vi "Read Video.vi"(6 "error in (no error)":errorcluster, 9 "input cluster":T6={"Video Resolution"=enum."FREENECT_RESOLUTION_LOW", "Video Format"=enum."FREENECT_VIDEO_RGB", "Depth Format"=enum."FREENECT_DEPTH_11BIT", "Depth Resolution"=enum."FREENECT_RESOLUTION_LOW"}) -> (0 "error out":errorcluster, 1 "raw data":u32[][](array[numeric]), 2 "Distance O":dbl, 3 "RGB image":picture, 4 "y":dbl, 5 "x":dbl)   [LabVIEW 2015]
uses:
  Video Resolution Control.ctl
  Video Format Control.ctl
  Depth Resolution Control.ctl
  <vilib>/picture/picture.llb/Draw True-Color Pixmap.vi
  libkinect_wrapper.dll
  <vilib>/vision/NI_Vision_Development_Module.lvlib
panel:
  out "Distance H":dbl
  out "Width":dbl
  in  "Number of Erosion":i32=2
  out "Centroid":cluster{"X Centroid":sgl, "Y Centroid":sgl} {"Y Centroid" format="%.2f"; "X Centroid" format="%.2f"}
  out "Largest Particle Image":T1(plugin-control)
  in  "HSL Ranges":T2={"Hue Range"={"Lower value"=80, "Upper value"=255}, "Sat Range"={"Lower value"=0, "Upper value"=30}, "Luma Range"={"Lower value"=0, "Upper value"=60}}
  out "error out 3":errorcluster
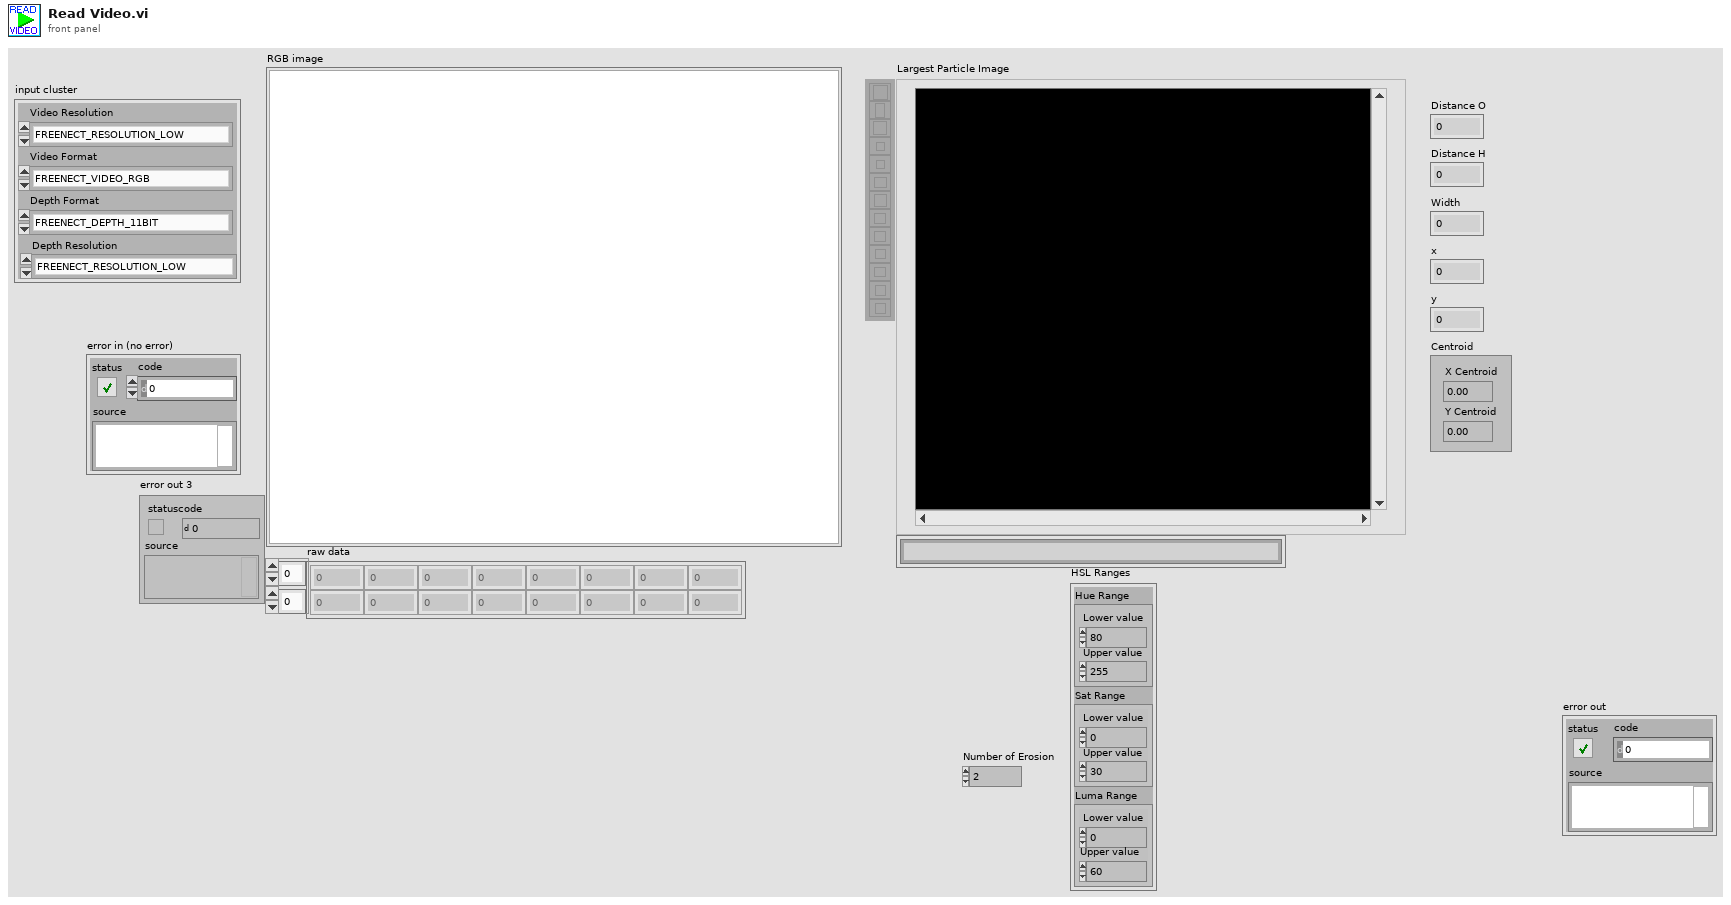
[diagram p1: front panel]
types:
  T1 = typedef "IMAQ Image.ctl" = refnum<image>
  T2 = cluster{"Hue Range":cluster{"Lower value":i32, "Upper value":i32}, "Sat Range":cluster{"Lower value":i32, "Upper value":i32}, "Luma Range":cluster{"Lower value":i32, "Upper value":i32}}
  T3 = typedef "Video Resolution Control.ctl" = enum32{"FREENECT_RESOLUTION_LOW", "FREENECT_RESOLUTION_MEDIUM", "FREENECT_RESOLUTION_HIGH"}
  T4 = typedef "Video Format Control.ctl" = enum32{"FREENECT_VIDEO_RGB", "FREENECT_VIDEO_BAYER", "FREENECT_VIDEO_IR_8BIT", "FREENECT_VIDEO_IR_10BIT", "FREENECT_VIDEO_IR_10BIT_PACKED", "FREENECT_VIDEO_YUV_RGB", "FREENECT_VIDEO_YUV_RAW"}
  T5 = typedef "Depth Resolution Control.ctl" = enum16{"FREENECT_RESOLUTION_TINY", "FREENECT_RESOLUTION_LOW", "FREENECT_RESOLUTION_MEDIUM"}
  T6 = cluster{"Video Resolution":T3, "Video Format":T4, "Depth Format":enum32{"FREENECT_DEPTH_11BIT", "FREENECT_DEPTH_10BIT", "FREENECT_DEPTH_11BIT_PACKED", "FREENECT_DEPTH_10BIT_PACKED", "FREENECT_DEPTH_REGISTERED", "FREENECT_DEPTH_MM"}, "Depth Resolution":T5}
  T7 = cluster{"X Size":i32, "Y Size":i32, "Order #":i32}
  T8 = typedef "Image Type" = u32
  T9 = cluster{"Area":dbl, "Number of Holes":dbl, "Bounding Rect":cluster{"Left":dbl, "Top":dbl, "Right":dbl, "Bottom":dbl}, "Center of Mass":cluster{"X":dbl, "Y":dbl}, "Orientation":dbl, "Dimensions":cluster{"Width":dbl, "Height":dbl}}[]
  T10 = cluster{"Area":dbl, "Number of Holes":dbl, "Bounding Rect":cluster{"Left":dbl, "Top":dbl, "Right":dbl, "Bottom":dbl}, "Center of Mass":cluster{"X":dbl, "Y":dbl}, "Orientation":dbl, "Dimensions":cluster{"Width":dbl, "Height":dbl}}
  T11 = cluster{"Left":dbl, "Top":dbl, "Right":dbl, "Bottom":dbl}
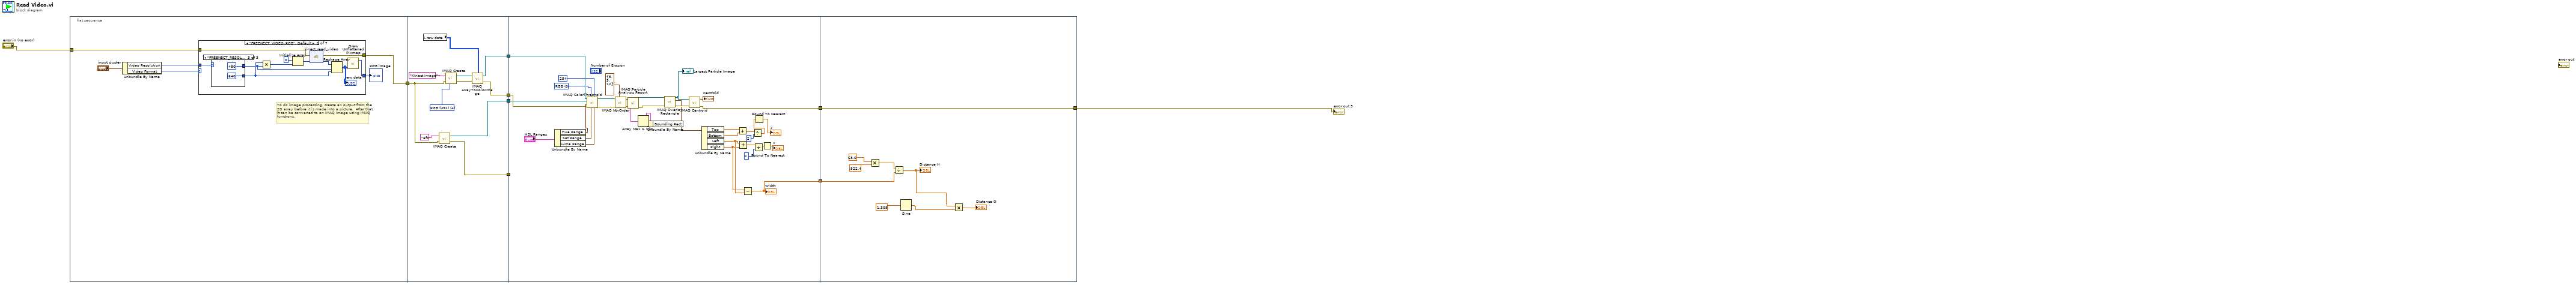
[diagram p0: block diagram]
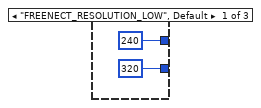
[diagram p2: hidden frame]
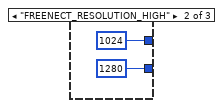
[diagram p3: hidden frame]
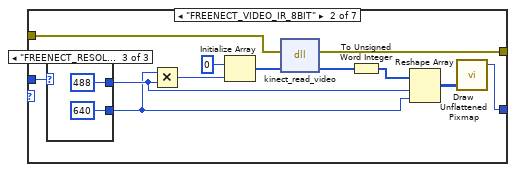
[diagram p4: hidden frame]
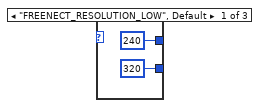
[diagram p5: hidden frame]
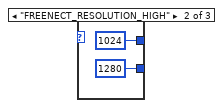
[diagram p6: hidden frame]
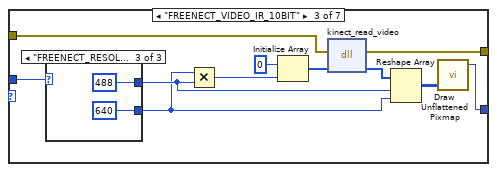
[diagram p7: hidden frame]
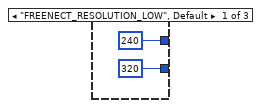
[diagram p8: hidden frame]
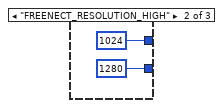
[diagram p9: hidden frame]
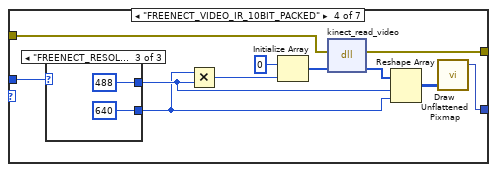
[diagram p10: hidden frame]
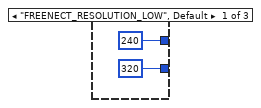
[diagram p11: hidden frame]
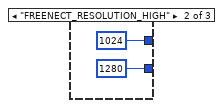
[diagram p12: hidden frame]
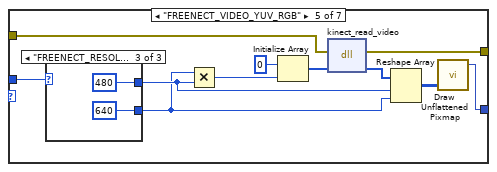
[diagram p13: hidden frame]
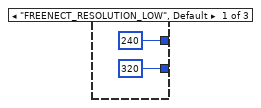
[diagram p14: hidden frame]
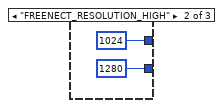
[diagram p15: hidden frame]
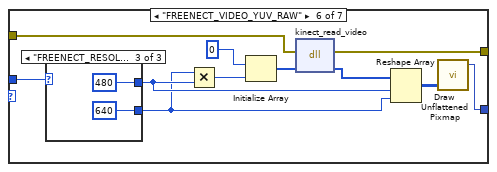
[diagram p16: hidden frame]
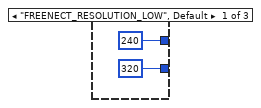
[diagram p17: hidden frame]
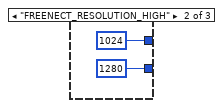
[diagram p18: hidden frame]
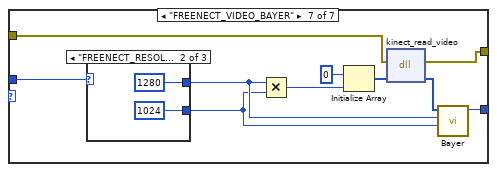
[diagram p19: hidden frame]
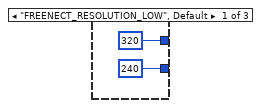
[diagram p20: hidden frame]
diagram:
  n1 = flat-sequence {
    tunnel: [w12] -> w9
    tunnel: "error in (no error)" -> [w10]
    tunnel: w9 -> [w136]
    tunnel: [w143] -> w7
    tunnel: [w140] -> w6
    tunnel: [w138] -> w5
    tunnel: [w135] -> w3
    tunnel: w7 -> [w168]
    tunnel: w6 -> [w157]
    tunnel: w5 -> [w169]
    tunnel: [w173] -> w4
    tunnel: w3 -> [_]
    tunnel: [w150] -> w1
    tunnel: w4 -> [w190]
    tunnel: [w190] -> w2
    tunnel: w1 -> [w186]
    frame #0 {
      # "To do image processing, create an output from the 2D array before it is made into a picture.  After that, it can be converted to an IMAQ image using IMAQ functions."
      n2 = Unbundle By Name("input cluster") -> ("Video Resolution"=w13:T3, "Video Format"=w14:T4)
      n3 = case shown="\"FREENECT_VIDEO_RGB\", Default" w14 {
        tunnel: w13 -> [w26 w36 w51 w70 w95 w112 w121]
        tunnel: [w22 w38 w53 w72 w89 w103 w122] -> w11
        tunnel: w10 -> [w21 w37 w52 w71 w88 w108 w124]
        tunnel: [w20 w39 w54 w73 w87 w107 w123] -> w12
        frame "FREENECT_VIDEO_RGB", Default {
          n4 = case shown="\"FREENECT_RESOLUTION_MEDIUM\"" w26 {
            tunnel: [240 1024 480] -> w19
            tunnel: [320 1280 640] -> w18
            frame "FREENECT_RESOLUTION_LOW", Default {
            }
            frame "FREENECT_RESOLUTION_HIGH" {
            }
            frame "FREENECT_RESOLUTION_MEDIUM" {
            }
          }
          n5 = Multiply(x=w18, y=w19) -> (x*y=w25:i32)
          n6 = Initialize Array(u32 0 ("U32"), w25) -> (w24:u32[])
          n7 = dll-call lib="libkinect_wrapper.*" fn="kinect_read_video"(error in=w21, "video"=w24) -> (error out=w20:errorcluster, "video"=w17:u32[])  [unwired: 3 in, 1 out]
          n8 = Reshape Array(w17, w19, w18) -> (w16:u32[][])
          "raw data" <- w16
          n9 = call-poly <vilib>:"Draw Unflattened Pixmap.vi"("data (RGB format)"=w16) -> ("new picture"=w22:picture)  [unwired: 8 in]
        }
        frame "FREENECT_VIDEO_IR_8BIT" {
          n10 = case shown="\"FREENECT_RESOLUTION_MEDIUM\"" w36 {
            tunnel: [240 1024 488] -> w41
            tunnel: [320 1280 640] -> w40
            frame "FREENECT_RESOLUTION_LOW", Default {
            }
            frame "FREENECT_RESOLUTION_HIGH" {
            }
            frame "FREENECT_RESOLUTION_MEDIUM" {
            }
          }
          n11 = Multiply(x=w40, y=w41) -> (x*y=w44:i32)
          n12 = Initialize Array(u8 0 ("U32"), w44) -> (w43:u8[])
          n13 = dll-call lib="libkinect_wrapper.*" fn="kinect_read_video"(error in=w37, "video"=w43) -> (error out=w39:errorcluster, "video"=w35:u8[])  [unwired: 3 in, 1 out]
          n14 = To Unsigned Word Integer(number=w35) -> (unsigned 16bit integer=w34:u16[])
          n15 = Reshape Array(w34, w41, w40) -> (w33:u16[][])
          n16 = call-poly <vilib>:"Draw Unflattened Pixmap.vi"("data (RGB format)"=w33) -> ("new picture"=w38:picture)  [unwired: 8 in]
        }
        frame "FREENECT_VIDEO_IR_10BIT" {
          n17 = case shown="\"FREENECT_RESOLUTION_MEDIUM\"" w51 {
            tunnel: [240 1024 488] -> w56
            tunnel: [320 1280 640] -> w55
            frame "FREENECT_RESOLUTION_LOW", Default {
            }
            frame "FREENECT_RESOLUTION_HIGH" {
            }
            frame "FREENECT_RESOLUTION_MEDIUM" {
            }
          }
          n18 = Multiply(x=w55, y=w56) -> (x*y=w61:i32)
          n19 = Initialize Array(u16 0 ("U32"), w61) -> (w60:u16[])
          n20 = dll-call lib="libkinect_wrapper.*" fn="kinect_read_video"(error in=w52, "video"=w60) -> (error out=w54:errorcluster, "video"=w58:u16[])  [unwired: 3 in, 1 out]
          n21 = Reshape Array(w58, w56, w55) -> (w57:u16[][])
          n22 = call-poly <vilib>:"Draw Unflattened Pixmap.vi"("data (RGB format)"=w57) -> ("new picture"=w53:picture)  [unwired: 8 in]
        }
        frame "FREENECT_VIDEO_IR_10BIT_PACKED" {
          n23 = case shown="\"FREENECT_RESOLUTION_MEDIUM\"" w70 {
            tunnel: [240 1024 488] -> w75
            tunnel: [320 1280 640] -> w74
            frame "FREENECT_RESOLUTION_LOW", Default {
            }
            frame "FREENECT_RESOLUTION_HIGH" {
            }
            frame "FREENECT_RESOLUTION_MEDIUM" {
            }
          }
          n24 = Multiply(x=w74, y=w75) -> (x*y=w78:i32)
          n25 = Initialize Array(u16 0 ("U32"), w78) -> (w77:u16[])
          n26 = dll-call lib="libkinect_wrapper.*" fn="kinect_read_video"(error in=w71, "video"=w77) -> (error out=w73:errorcluster, "video"=w69:u16[])  [unwired: 3 in, 1 out]
          n27 = Reshape Array(w69, w75, w74) -> (w68:u16[][])
          n28 = call-poly <vilib>:"Draw Unflattened Pixmap.vi"("data (RGB format)"=w68) -> ("new picture"=w72:picture)  [unwired: 8 in]
        }
        frame "FREENECT_VIDEO_YUV_RGB" {
          n29 = case shown="\"FREENECT_RESOLUTION_MEDIUM\"" w95 {
            tunnel: [240 1024 480] -> w86
            tunnel: [320 1280 640] -> w85
            frame "FREENECT_RESOLUTION_LOW", Default {
            }
            frame "FREENECT_RESOLUTION_HIGH" {
            }
            frame "FREENECT_RESOLUTION_MEDIUM" {
            }
          }
          n30 = Multiply(x=w85, y=w86) -> (x*y=w94:i32)
          n31 = Initialize Array(u32 0 ("U32"), w94) -> (w93:u32[])
          n32 = dll-call lib="libkinect_wrapper.*" fn="kinect_read_video"(error in=w88, "video"=w93) -> (error out=w87:errorcluster, "video"=w91:u32[])  [unwired: 3 in, 1 out]
          n33 = Reshape Array(w91, w86, w85) -> (w90:u32[][])
          n34 = call-poly <vilib>:"Draw Unflattened Pixmap.vi"("data (RGB format)"=w90) -> ("new picture"=w89:picture)  [unwired: 8 in]
        }
        frame "FREENECT_VIDEO_YUV_RAW" {
          n35 = case shown="\"FREENECT_RESOLUTION_MEDIUM\"" w112 {
            tunnel: [240 1024 480] -> w106
            tunnel: [320 1280 640] -> w105
            frame "FREENECT_RESOLUTION_LOW", Default {
            }
            frame "FREENECT_RESOLUTION_HIGH" {
            }
            frame "FREENECT_RESOLUTION_MEDIUM" {
            }
          }
          n36 = Multiply(x=w105, y=w106) -> (x*y=w111:i32)
          n37 = Initialize Array(u16 0 ("U32"), w111) -> (w110:u16[])
          n38 = dll-call lib="libkinect_wrapper.*" fn="kinect_read_video"(error in=w108, "video"=w110) -> (error out=w107:errorcluster, "video"=w104:u16[])  [unwired: 3 in, 1 out]
          n39 = Reshape Array(w104, w106, w105) -> (w102:u16[][])
          n40 = call-poly <vilib>:"Draw Unflattened Pixmap.vi"("data (RGB format)"=w102) -> ("new picture"=w103:picture)  [unwired: 8 in]
        }
        frame "FREENECT_VIDEO_BAYER" {
          n41 = case shown="\"FREENECT_RESOLUTION_HIGH\"" w121 {
            tunnel: [320 1280 640] -> w120
            tunnel: [240 1024 480] -> w119
            frame "FREENECT_RESOLUTION_LOW", Default {
            }
            frame "FREENECT_RESOLUTION_HIGH" {
            }
            frame "FREENECT_RESOLUTION_MEDIUM" {
            }
          }
          n42 = Multiply(x=w120, y=w119) -> (x*y=w128:i32)
          n43 = Initialize Array(u8 0, w128) -> (w127:u8[])
          n44 = dll-call lib="libkinect_wrapper.*" fn="kinect_read_video"(error in=w124, "video"=w127) -> (error out=w123:errorcluster, "video"=w126:u8[])  [unwired: 3 in, 1 out]
          n45 = call "Bayer.vi"("Height"=w119, "Width"=w120, "Array"=w126) -> ("new picture"=w122:picture)  [unwired: 8 in]
        }
      }
      "RGB image" <- w11
    }
    frame #1 {
      w137 = T8 4 items=["Grayscale (U8)", "Grayscale (I16)", "Grayscale (SGL)", "Complex (CSG)", "RGB (U32)", "HSL (U32)", "RGB (U64)", "Grayscale (U16)"] ("Image Type")
      n46 = local read "raw data"() -> (w141:u32[][])
      n47 = call "IMAQ Create"("Image Name"="afs", "error in (no error)"=w136) -> ("New Image"=w138:T1, "error out"=w135:errorcluster)  [unwired: 3 in]
      n48 = call "IMAQ Create"("Image Name"="Kinect image", "Image Type"=w137, "error in (no error)"=w136) -> ("New Image"=w145:T1, "error out"=w144:errorcluster)  [unwired: 2 in]
      n49 = call "IMAQ ArrayToColorImage"("Image Pixels (U32)"=w141, "Image"=w145, "error in (no error)"=w144) -> ("Image Out"=w140:T1, "error out"=w143:errorcluster)  [unwired: 2 in]
    }
    frame #2 {
      w170 = u16 0 items=["RGB", "HSL", "HSV", "HSI"] ("Color Mode")
      n50 = Unbundle By Name("HSL Ranges") -> ("Hue Range"=w180:cluster{"Lower value":i32, "Upper value":i32}, "Sat Range"=w179:cluster{"Lower value":i32, "Upper value":i32}, "Luma Range"=w158:cluster{"Lower value":i32, "Upper value":i32})
      n51 = call "IMAQ ColorThreshold"("Blue or Luma or Val or Inten Range"=w158, "Replace Value"=254, "Green or Sat Range"=w179, "Color Mode"=w170, "error in (no error)"=w168, "Red or Hue Range"=w180, "Image Dst"=w169, "Image Src"=w157) -> ("error out"=w146:errorcluster, "Image Dst Out"=w147:T1)  [unwired: 2 in]
      n52 = call "IMAQ NthOrder"("Image Src"=w147, "Size & Order #"=T7 {"X Size"=5, "Y Size"=5, "Order #"=12}, "error in (no error)"=w146) -> ("Image Dst Out"=w155:T1, "error out"=w154:errorcluster)  [unwired: 4 in]
      n53 = call "IMAQ Particle Analysis Report"("error in (no error)"=w154, "Image"=w155) -> ("error out"=w176:errorcluster, "Particle Reports (Pixels)"=w177:T9, "Image Out (duplicate)"=w156:T1)  [unwired: 4 in, 3 out]
      n54 = Array Max & Min(array=w177) -> (max value=w175:T10)  [unwired: 3 out]
      n55 = Unbundle By Name(w175) -> ("Bounding Rect"=w167:T11)
      n56 = call "IMAQ Overlay Rectangle"("error in (no error)"=w176, "Rectangle"=w167, "Image"=w156) -> ("error out"=w174:errorcluster, "Image Out"=w172:T1)  [unwired: 7 in]
      "Largest Particle Image" <- w172
      n57 = call "IMAQ Centroid"("error in (no error)"=w174, "Image"=w172) -> ("error out"=w173:errorcluster, "Centroid"=→"Centroid":cluster{"X Centroid":sgl, "Y Centroid":sgl})  [unwired: 2 in]
      n58 = Unbundle By Name(w167) -> ("Top"=w149:dbl, "Bottom"=w148:dbl, "Left"=w152:dbl, "Right"=w151:dbl)
      n59 = Add(x=w149, y=w148) -> (x+y=w165:dbl)
      n60 = Add(x=w152, y=w151) -> (x+y=w166:dbl)
      n61 = Subtract(x=w151, y=w152) -> (x-y=w150:dbl)
      "Width" <- w150
      n62 = Divide(x=w165, y=2) -> (x/y=w159:dbl)
      n63 = Divide(x=w166, y=2) -> (x/y=w162:dbl)
      n64 = Round To Nearest(number=w159) -> (nearest integer value=→"y":dbl)
      n65 = Round To Nearest(number=w162) -> (nearest integer value=→"x":dbl)
    }
    frame #3 {
      n66 = Multiply(x=68.0, y=522.4) -> (x*y=w187:dbl)
      n67 = Divide(x=w187, y=w186) -> (x/y=w184:dbl)
      "Distance H" <- w184
      n68 = Sine(x=1.309) -> (sin(x)=w183:dbl)
      n69 = Multiply(x=w184, y=w183) -> (x*y=→"Distance O":dbl)
    }
  }
  "error out 3" <- w2
